vi "Set TDF - Parameters.vi"(0 "reference in":refnum<class "GSwFormDSP.lvclass">, 5 "error in (no error)":errorcluster, 7 "TDF Parameters":T1={"Filter"=enum."Lowpass", "Type:"=enum."Elliptic", "LP cutoff freq"=600.0, "HP cutoff freq"=100.0, "Order"=8, "passband ripple (dB)"=0.1, "stopband attenuation (dB)"=60.0, "Phaseless Filter"=TRUE, "Include Fade IN and OUT"=FALSE} {"stopband attenuation (dB)" format="%.2f"; "passband ripple (dB)" format="%.2f"; "HP cutoff freq" format="%#.3f"; "LP cutoff freq" format="%#.3f"}) -> (13 "Cut Off Freq. Coerced?":bool, 14 "reference out":refnum<class "GSwFormDSP.lvclass">, 19 "error out":errorcluster)   [LabVIEW 2020, in "GSwFormDSP.lvclass"]
uses:
  GSwFormDSP.lvclass
  functions/TDF Parameters.ctl
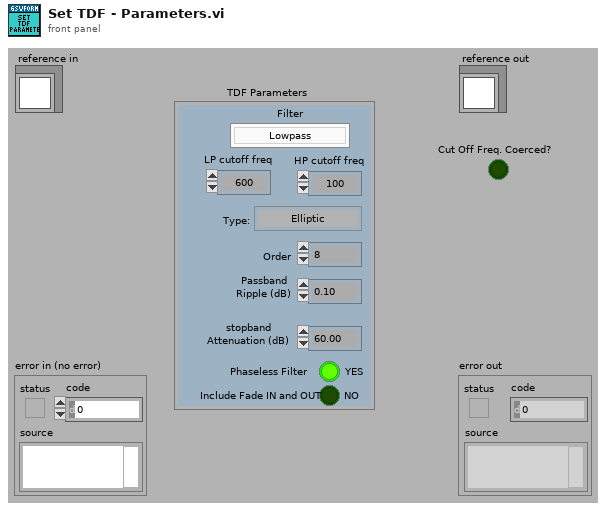
[diagram p1: front panel]
types:
  T1 = typedef "GSwFormDSP.lvclass/TDF Parameters.ctl" = cluster{"Filter":enum32{"Lowpass", "Highpass", "Bandpass", "Bandstop"}, "Type:":enum16{"Butterworth", "Chebyshev", "Inv Chebyshev", "Elliptic", "Bessel"}, "LP cutoff freq":dbl, "HP cutoff freq":dbl, "Order":i32, "passband ripple (dB)":dbl, "stopband attenuation (dB)":dbl, "Phaseless Filter":bool, "Include Fade IN and OUT":bool}
  T2 = typedef "GSwFormDSP.lvclass/ObjectAttributesRef.ctl" = refnum<data-value>
  T3 = typedef "GSwFormDSP.lvclass/ObjectAttributes.ctl" = cluster{"Wform Ref":refnum<data-value>, "Nb Signals":i32, "Spectral Function Parameters":T4, "FFT":waveform(cdb)[], "Nb FFT":i32, "Nb Averages":i32[], "Reference Indexes":i32[], "Response Indexes":i32[], "Coherence":waveform(dbl)[], "TDF Parameters":T1, "DAQ":cluster{"Duration (sec)":dbl, "Buffer Size (Samples)":i32, "Offset (Samples)":i32}, "Filter Impulse Response (TDF)":waveform(dbl), "Sound Playback":T6}
  T4 = typedef "GSwFormDSP.lvclass/Spectral Parameters.ctl" = cluster{"Frequency resolution (Hz)":dbl, "Overlap":dbl, "Window":T5}
  T5 = typedef "NI_AALPro.lvlib/windowTd.ctl" = u32
  T6 = typedef "GSwFormDSP.lvclass/Sound Playback.ctl" = cluster{"Timer start (ms)":u32, "task ID":T7, "Cursor Init Location (s)":dbl, "SC Volume":dbl}
  T7 = typedef "Sound Output Task ID.ctl" = u32
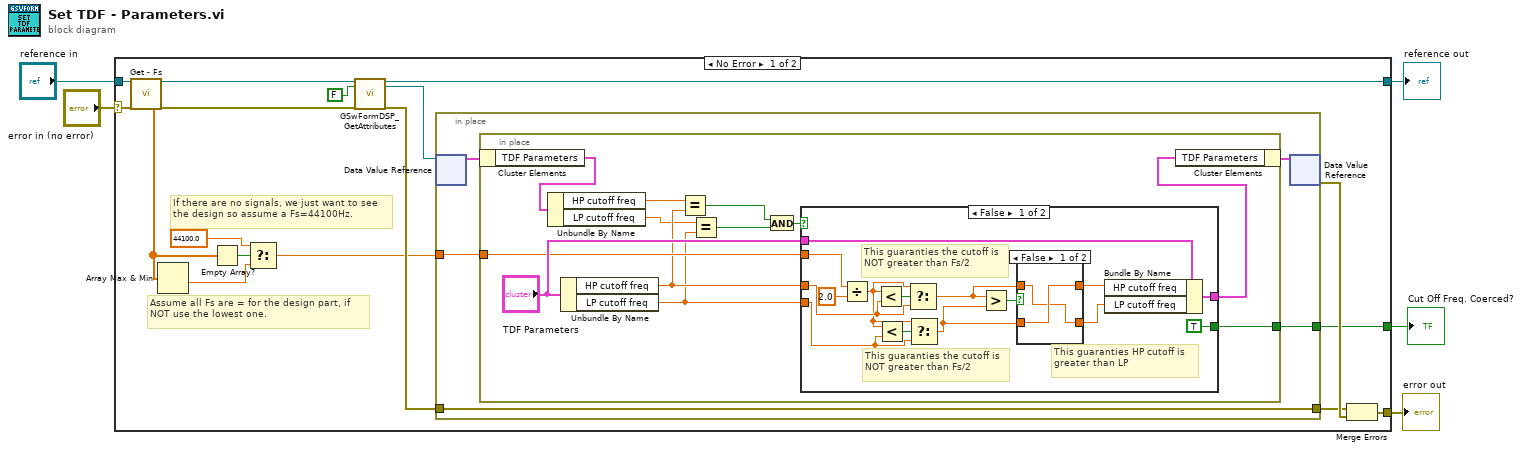
[diagram p0: block diagram]
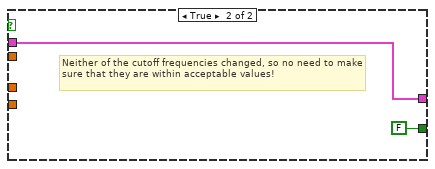
[diagram p3: hidden frame]
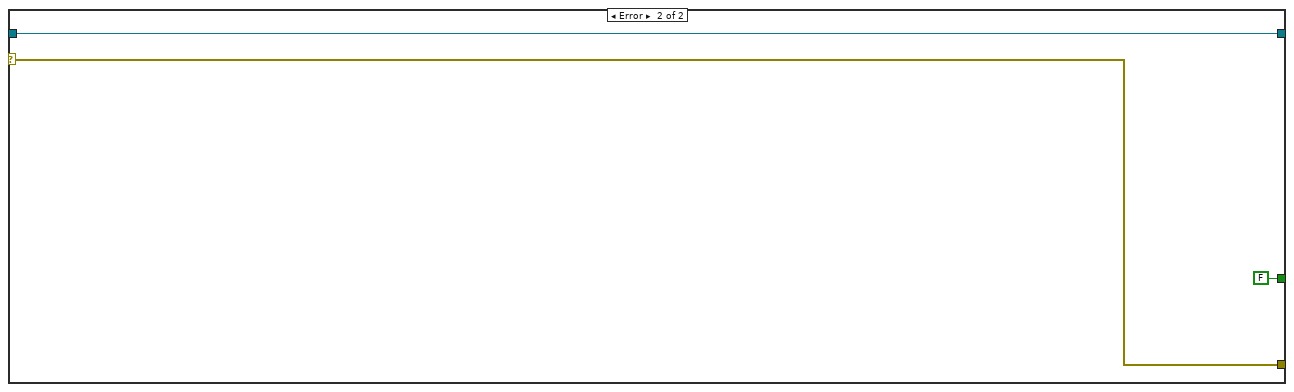
[diagram p4: hidden frame]
diagram:
  n1 = case shown="No Error" "error in (no error)" {
    selector: "error in (no error)" -> [w10 w63]
    tunnel: [w22 w63] -> w4
    tunnel: [w17 w62] -> w2
    tunnel: "reference in" -> [w11 w62]
    tunnel: [w6 FALSE] -> w1
    frame No Error {
      # "If there are no signals, we just want to see the design so assume a Fs=44100Hz."
      # "Assume all Fs are = for the design part, if NOT use the lowest one."
      n2 = call-dynamic "Get - Fs.vi"("reference in"=w11, "error in (no error)"=w10) -> ("Signals Fs"=w15:dbl[], "reference in"=w9:refnum<class "GSwFormDSP.lvclass">, "error out"=w8:errorcluster)  [unwired: 14 in, 1 out]
      n3 = Array Max & Min(array=w15) -> (min value=w13:dbl)  [unwired: 3 out]
      n4 = Empty Array?(array=w15) -> (empty?=w14:bool)
      n5 = Select(t=44100.0, s=w14, f=w13) -> (s? t:f=w7:dbl)
      n6 = call "GSwFormDSP_GetAttributes.vi"("reference in"=w9, "return data? (T)"=FALSE, "error in (no error)"=w8) -> ("reference out"=w17:refnum<class "GSwFormDSP.lvclass">, "attributes ref"=w16:T2, "error out"=w18:errorcluster)  [unwired: 13 in, 1 out]
      n7 = in-place {
        in-place-border: w18 -> [w25]
        in-place-border: [w25] -> w20
        in-place-border: w7 -> [w24]
        in-place-border: [w23] -> w6
        n8 = in-place-dvr #1(w16) -> (w26:T3)  [unwired: 1 out]
        n9 = in-place {
          in-place-border: w24 -> [w38]
          in-place-border: [w28] -> w23
          n10 = in-place-cluster #2(w26) -> ("TDF Parameters"=w37:T1)
          n11 = Unbundle By Name(w37) -> ("HP cutoff freq"=w34:dbl, "LP cutoff freq"=w32:dbl)
          n12 = Unbundle By Name("TDF Parameters") -> ("HP cutoff freq"=w33:dbl, "LP cutoff freq"=w31:dbl)
          n13 = Equal?(x=w34, y=w33) -> (x = y?=w29:bool)
          n14 = Equal?(x=w32, y=w31) -> (x = y?=w30:bool)
          n15 = And(x=w29, y=w30) -> (x .and. y?=w36:bool)
          n16 = case shown="False" w36 {
            tunnel: w31 -> [w49 _]
            tunnel: w33 -> [w48 _]
            tunnel: "TDF Parameters" -> [w43 w60]
            tunnel: [w42 w60] -> w35
            tunnel: w38 -> [w41 _]
            tunnel: [TRUE FALSE] -> w28
            frame False {
              # "This guaranties HP cutoff is greater than LP"
              # "This guaranties the cutoff is NOT greater than Fs/2"
              # "This guaranties the cutoff is NOT greater than Fs/2"
              n17 = Divide(x=w41, y=2.0) -> (x/y=w44:dbl)
              n18 = Less?(x=w44, y=w48) -> (x < y?=w46:bool)
              n19 = Less?(x=w44, y=w49) -> (x < y?=w45:bool)
              n20 = Select(t=w44, s=w46, f=w48) -> (s? t:f=w52:dbl)
              n21 = Select(t=w44, s=w45, f=w49) -> (s? t:f=w54:dbl)
              n22 = Greater?(x=w52, y=w54) -> (0:w50:bool)
              n23 = case shown="False" w50 {
                tunnel: [w56 w58] -> w51
                tunnel: w52 -> [w55 w58]
                tunnel: [w55 w57] -> w53
                tunnel: w54 -> [w56 w57]
                frame False {
                }
                frame True {
                }
              }
              n24 = Bundle By Name(cluster=w43, "HP cutoff freq"=w51, "LP cutoff freq"=w53) -> (w42:T1)
            }
            frame True {
              # "Neither of the cutoff frequencies changed, so no need to make sure that they are within acceptable values!"
            }
          }
          n25 = in-place-cluster #2("TDF Parameters"=w35) -> (w27:T3)
        }
        n26 = in-place-dvr #1(w27) -> (w21:errorcluster)  [unwired: 1 out]
      }
      n27 = Merge Errors(w20, w21) -> (w22:errorcluster)
    }
    frame Error {
    }
  }
  "error out" <- w4
  "reference out" <- w2
  "Cut Off Freq. Coerced?" <- w1
